vi "GPS参数配置.vi"() -> ()   [LabVIEW 2016, in "环境动力监测库.lvlib" / "NMEA.lvlib"]
uses:
  NMEA.lvlib
panel:
  in  "纬度":dbl
  in  "经度":dbl
  in  "手动设置定位":bool caption="定位自动获取OFF/手动设置ON"
  in  "移位报警设定值":dbl=1000.0
  # "GPS参数配置"
  # "米"
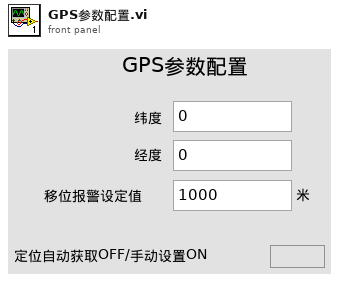
[diagram p1: front panel]
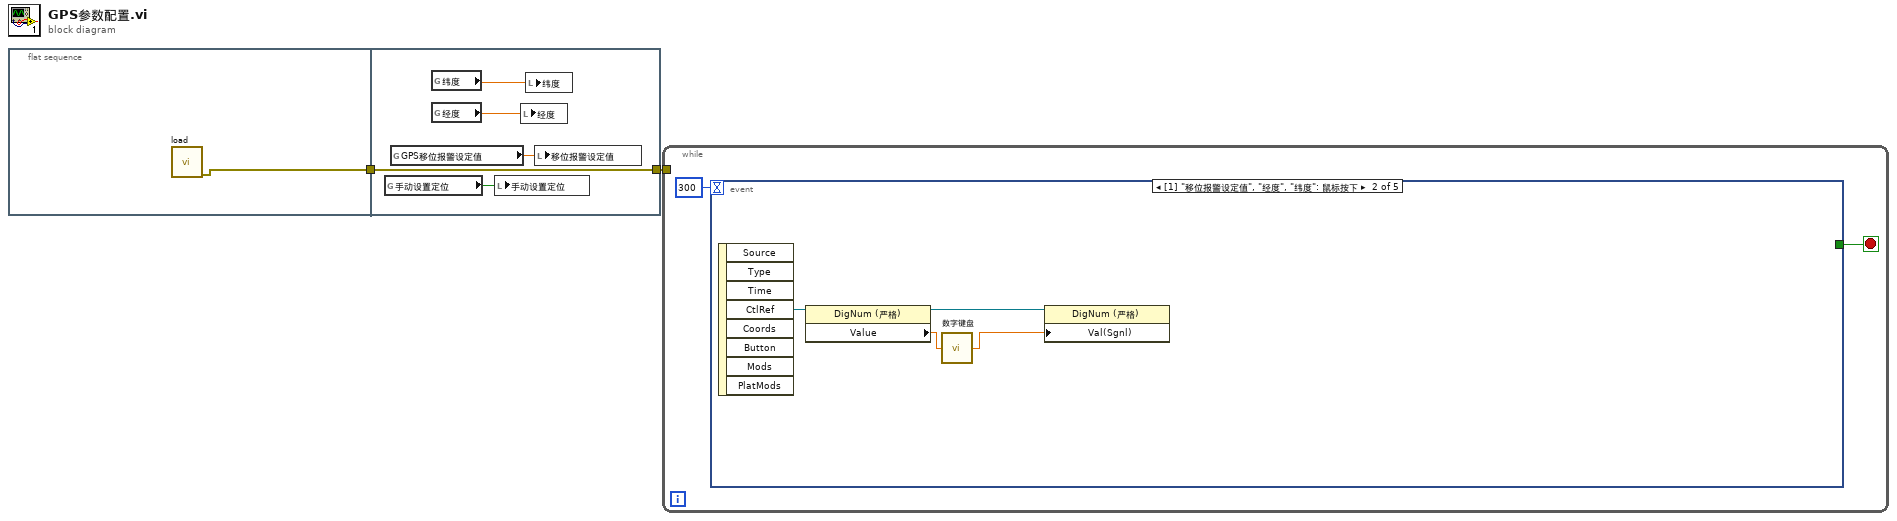
[diagram p0: block diagram]
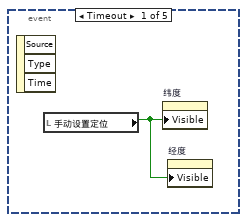
[diagram p2: hidden frame]
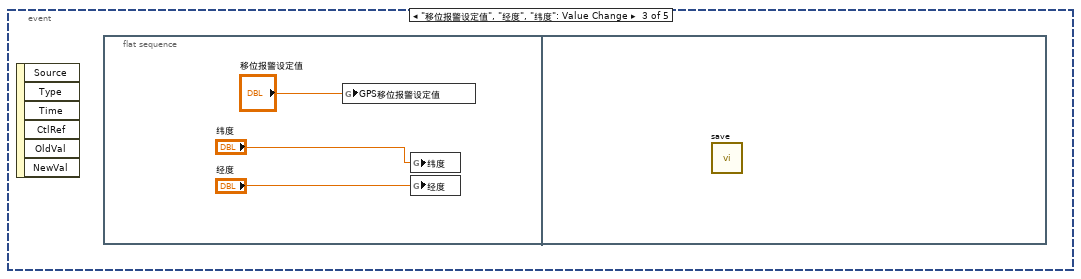
[diagram p3: hidden frame]
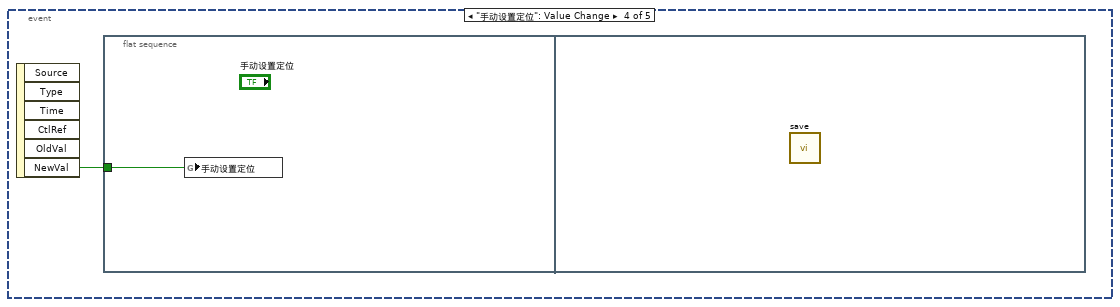
[diagram p4: hidden frame]
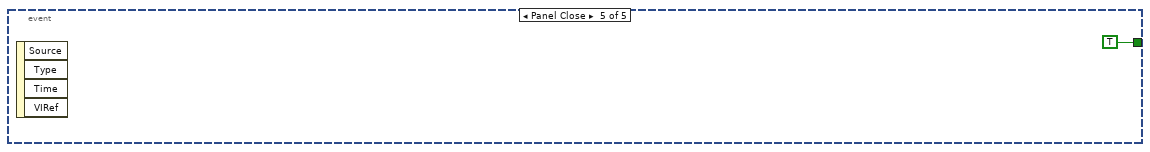
[diagram p5: hidden frame]
diagram:
  n1 = flat-sequence {
    tunnel: [w3] -> w2
    tunnel: [w8] -> w1
    tunnel: w2 -> [w8]
    frame #0 {
      n2 = call "load.vi"() -> ("error out"=w3:errorcluster)  [unwired: 11 in]
    }
    frame #1 {
      n3 = global read "断电保存全局变量.vi" "手动设置定位"() -> (w7:bool)
      n4 = global read "断电保存全局变量.vi" "GPS移位报警设定值"() -> (w5:dbl)
      n5 = global read "断电保存全局变量.vi" "纬度"() -> (w6:dbl)
      n6 = global read "断电保存全局变量.vi" "经度"() -> (w4:dbl)
      n7 = local write "手动设置定位"(w7) -> ()
      n8 = local write "经度"(w4) -> ()
      n9 = local write "纬度"(w6) -> ()
      n10 = local write "移位报警设定值"(w5) -> ()
    }
  }
  n11 = while {
    tunnel: w1 -> [_]
    stop <- w10 stop-if-true
    n12 = event shown="[1] \"移位报警设定值\", \"经度\", \"纬度\": 鼠标按下" {
      selector: _ -> [_ _ _ _ _]
      dyn-events: _ -> [_ _ _ _ _]
      timeout: 300 -> [_ _ _ _ _]
      tunnel: [_ _ _ _ TRUE] -> w10
      event Timeout {
        n13 = event-data() -> ()  [unwired: 1 in, 3 out]
        n14 = local read "手动设置定位"() -> (w11:bool)
        n15 = property on="纬度" class="DigNum (严格)"("Visible"=w11) -> ()  [unwired: 2 in, 2 out]
        n16 = property on="经度" class="DigNum (严格)"("Visible"=w11) -> ()  [unwired: 2 in, 2 out]
      }
      event "移位报警设定值", "经度", "纬度": Mouse Down {
        n17 = event-data() -> ("CtlRef"=w12:refnum<vi>)  [unwired: 1 in, 7 out]
        n18 = property class="DigNum (严格)"(reference=w12) -> (reference out=w14:refnum<vi>, "Value"=w15:dbl)  [unwired: 1 in, 1 out]
        n19 = call "数字键盘.vi"("OldNumber"=w15) -> ("NewNumber"=w13:sgl)
        n20 = property class="DigNum (严格)"(reference=w14, "Val(Sgnl)"=w13) -> ()  [unwired: 1 in, 2 out]
      }
      event "移位报警设定值", "经度", "纬度": Value Change {
        n21 = event-data() -> ()  [unwired: 1 in, 6 out]
        n22 = flat-sequence {
          frame #0 {
            n23 = global write "断电保存全局变量.vi" "GPS移位报警设定值"("移位报警设定值") -> ()
            n24 = global write "断电保存全局变量.vi" "纬度"("纬度") -> ()
            n25 = global write "断电保存全局变量.vi" "经度"("经度") -> ()
          }
          frame #1 {
            n26 = call "save.vi"() -> ()  [unwired: 11 in, 1 out]
          }
        }
      }
      event "手动设置定位": Value Change {
        n27 = event-data() -> ("NewVal"=w19:bool)  [unwired: 1 in, 5 out]
        n28 = flat-sequence {
          tunnel: w19 -> [w20]
          frame #0 {
            n29 = global write "断电保存全局变量.vi" "手动设置定位"(w20) -> ()
          }
          frame #1 {
            n30 = call "save.vi"() -> ()  [unwired: 11 in, 1 out]
          }
        }
      }
      event Panel Close {
        n31 = event-data() -> ()  [unwired: 1 in, 4 out]
      }
    }
  }
